vi "SaveDataIntoDB.vi"(8 "error in (no error)":errorcluster, 11 "ClashRoyale in":refnum<class "ClashRoyale.lvclass">) -> (0 "error out":errorcluster, 3 "ClashRoyale out":refnum<class "ClashRoyale.lvclass">)   [LabVIEW 2020, in "ClashRoyale.lvclass"]
uses:
  ClashRoyale.lvclass
  ClashRoyale.lvclass/ClashRoyale.ctl
  <vilib>/drjdpowell/SQLite Library/SQL Connection/Execute SQL (No results).vi
  <vilib>/drjdpowell/SQLite Library/SQLite.lvlib
  <vilib>/drjdpowell/SQLite Library/SQL Connection/Connection.lvclass
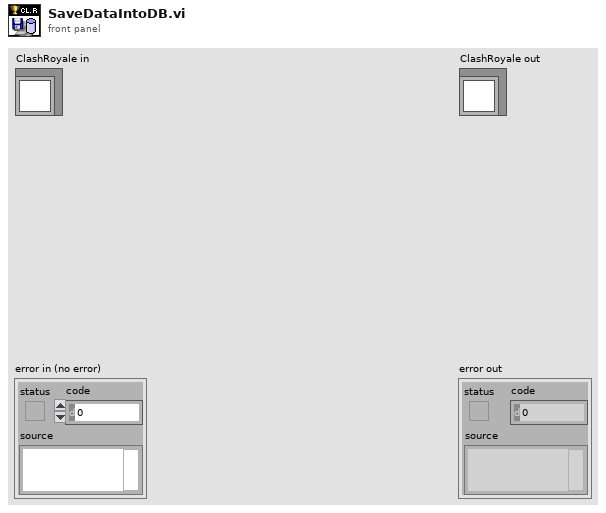
[diagram p1: front panel]
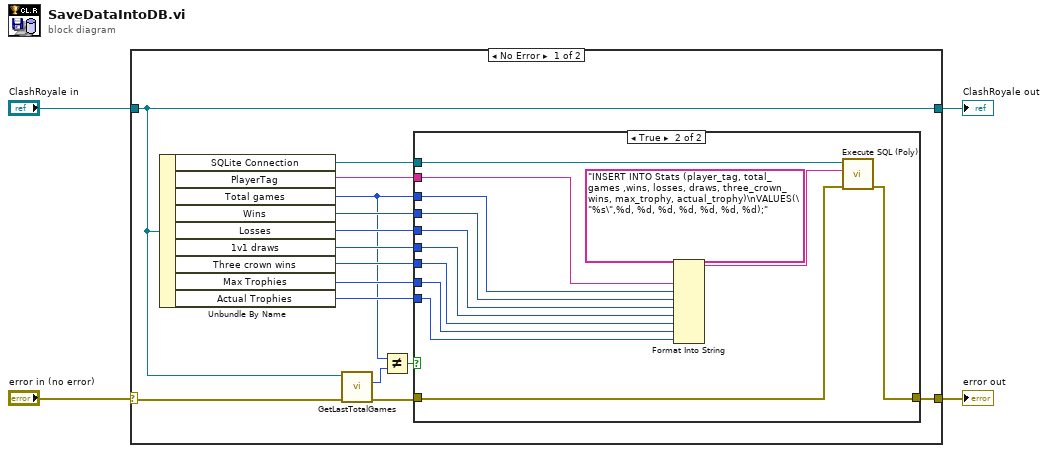
[diagram p0: block diagram]
diagram:
  n1 = case shown="No Error" "error in (no error)" {
    selector: "error in (no error)" -> [w9 w35]
    tunnel: [w13 w35] -> w3
    tunnel: [w10 w34] -> w1
    tunnel: "ClashRoyale in" -> [w10 w34]
    frame No Error {
      n2 = Unbundle By Name(w10) -> ("SQLite Connection"=w19:refnum<class "Connection.lvclass">, "PlayerTag"=w18:string, "Total games"=w6:u32, "Wins"=w17:u32, "Losses"=w16:u32, "1v1 draws"=w15:u32, "Three crown wins"=w14:u32, "Max Trophies"=w12:u32, "Actual Trophies"=w11:u32)
      n3 = call "GetLastTotalGames.vi"("error in (no error)"=w9, "ClashRoyale in"=w10) -> ("error out"=w8:errorcluster, "Last Total Games"=w7:i64)  [unwired: 7 in, 1 out]
      n4 = Not Equal?(x=w6, y=w7) -> (x != y?=w5:bool)
      n5 = case shown="True" w5 {
        tunnel: w19 -> [_ w33]
        tunnel: w18 -> [_ w31]
        tunnel: w6 -> [_ w30]
        tunnel: w17 -> [_ w29]
        tunnel: w16 -> [_ w28]
        tunnel: w15 -> [_ w27]
        tunnel: w14 -> [_ w26]
        tunnel: w8 -> [w20 w24]
        tunnel: [w20 w23] -> w13
        tunnel: w12 -> [_ w22]
        tunnel: w11 -> [_ w21]
        frame False {
          # "Pas de nouvelles parties jouées"
        }
        frame True {
          n6 = Format Into String(format string="INSERT INTO Stats (player_tag, total_games ,wins, losses, draws, three_crown_wins, max_trophy, actual_trophy)\nVALUES(\"%s\",%d, %d, %d, %d, %d, %d, %d);", w31, w30, w29, w28, w27, w26, w22, w21) -> (resulting string=w25:string)  [unwired: 2 in, 1 out]
          n7 = call-poly <vilib>:"Execute SQL (Poly).vi"("error in (no error)"=w24, "SQL"=w25, "SQLite Connection in"=w33) -> ("error out"=w23:errorcluster)  [unwired: 7 in, 1 out]
        }
      }
    }
    frame Error {
    }
  }
  "error out" <- w3
  "ClashRoyale out" <- w1
